vi "Test.vi"() -> ()   [LabVIEW 2017]
uses:
  libonnx_wrapper/libonnx_wrapper.lvlib
  postprocess_YOLOv8/postprocess_YOLOv8.lvlib
  libonnx_wrapper/TypeDef/IO.ctl
  libonnx_wrapper/TypeDef/Introspection.ctl
panel:
  out "Circles":cluster{"x":sgl, "y":sgl, "r":sgl}[](array[cluster])
  out "count":i32
  out "2D Picture":picture
  in  "BMP file path":path=path "/home/ivan/LabVIEWData/ONNX/LabVIEW_ONNX_YOLOv8/image_for_test/2005mmd_b2_1r_2005mmd_b2_var33.bmp"
  out "Metadata":string[][](table)
  out "Introspection Output":T1
  out "Introspection Input":T1
  in  "ONNX model path":path=path "/home/ivan/LabVIEWData/ONNX/LabVIEW_ONNX_YOLOv8/data/coins_detection.onnx"
  out "error out":errorcluster
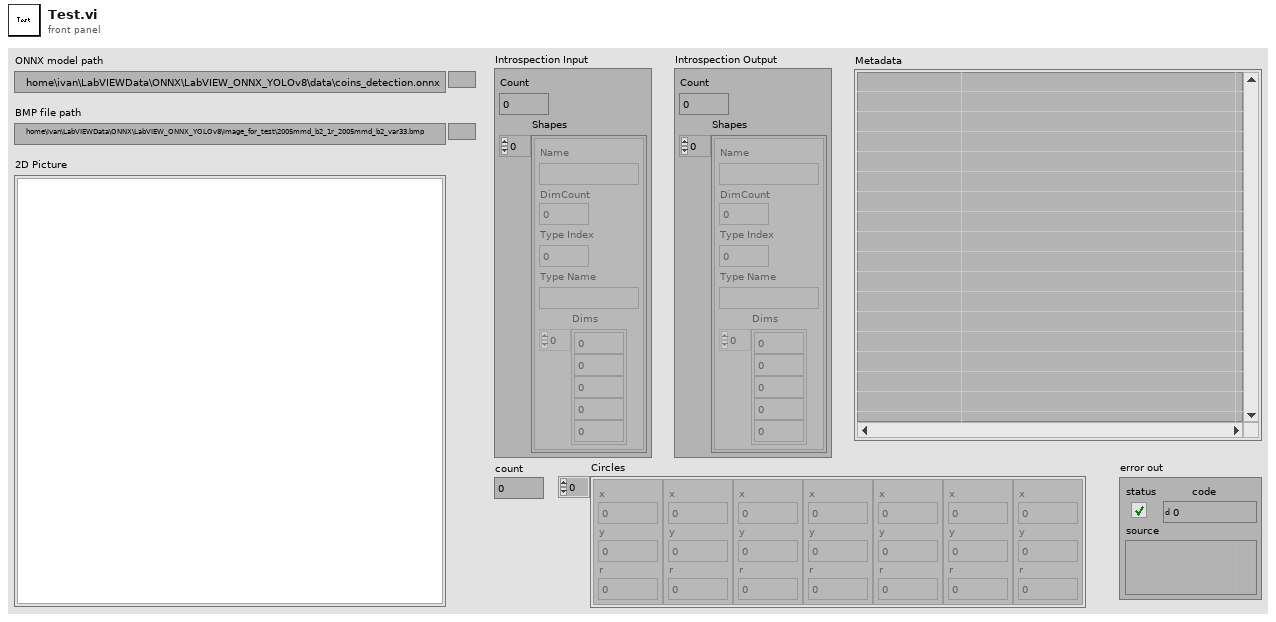
[diagram p1: front panel]
types:
  T1 = typedef "libonnx_wrapper.lvlib/Introspection.ctl" = cluster{"Count":i32, "Shapes":T2[]}
  T2 = typedef "libonnx_wrapper.lvlib/IO.ctl" = cluster{"Name":string, "DimCount":i32, "Type Index":i32, "Type Name":string, "Dims":i64[]}
  T3 = typedef "imagedata.ctl" = cluster{"image type":i32, "image depth":i32, "image":u8[], "mask":u8[], "colors":u32[], "Rectangle":cluster{"left":i16, "top":i16, "right":i16, "bottom":i16}}
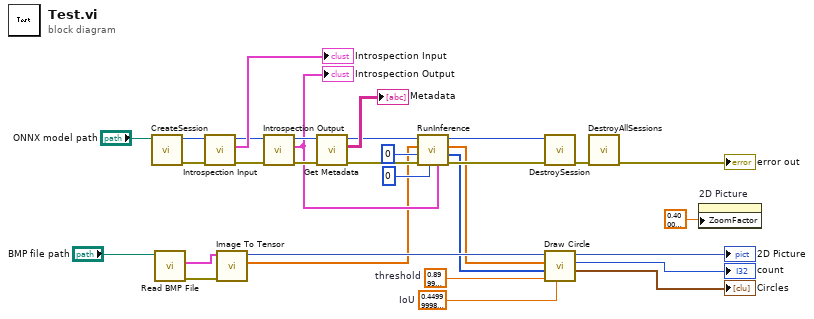
[diagram p0: block diagram]
diagram:
  w3 = sgl 0.45  # IoU
  w4 = sgl 0.9  # threshold
  n1 = call "CreateSession.vi"("ONNX model path"="ONNX model path") -> ("error out"=w14:errorcluster, "session id out"=w15:i32)  [unwired: 9 in]
  n2 = call <vilib>:"Read BMP File.vi"("path to BMP file"="BMP file path") -> ("error out"=w16:errorcluster, "image data"=w17:T3)  [unwired: 8 in, 1 out]
  n3 = call "Introspection Input.vi"("error in (no error)"=w14, "session id in"=w15) -> ("error out"=w27:errorcluster, "Introspection Input"=→"Introspection Input":T1, "session id out"=w28:i32)  [unwired: 7 in]
  n4 = call "Image To Tensor.vi"("error in (no error)"=w16, "image data"=w17) -> ("Data"=w7:sgl[], "image"=w11:picture)  [unwired: 7 in, 1 out]
  n5 = call "Introspection Output.vi"("error in (no error)"=w27, "session id in"=w28) -> ("error out"=w24:errorcluster, "Introspection Output"=w9:T1, "session id out"=w25:i32)  [unwired: 7 in]
  "Introspection Output" <- w9
  n6 = call "Get Metadata.vi"("error in (no error)"=w24, "session id in"=w25) -> ("error out"=w21:errorcluster, "Metadata"=→"Metadata":string[][], "session id out"=w22:i32)  [unwired: 7 in]
  n7 = call "RunInference.vi"("Introspection Output"=w9, "outputIndex"=0, "error in (no error)"=w21, "inputIndex"=0, "inputBuffer"=w7, "session id in"=w22) -> ("error out"=w13:errorcluster, "Dims"=w6:i64[], "outputBuffer"=w5:sgl[], "session id out"=w12:i32)  [unwired: 1 in, 1 out]
  n8 = call "DestroySession.vi"("error in (no error)"=w13, "session id in"=w12) -> ("error out"=w30:errorcluster)  [unwired: 8 in, 1 out]
  n9 = call "Draw Circle.vi"("IoU"=w3, "threshold"=w4, "dim"=w6, "data"=w5, "image in"=w11) -> ("Circles"=→"Circles":cluster{"x":sgl, "y":sgl, "r":sgl}[], "count"=→"count":i32, "image out"=→"2D Picture":picture)  [unwired: 4 in]
  n10 = call "DestroyAllSessions.vi"("error in (no error)"=w30) -> ("error out"=→"error out":errorcluster)  [unwired: 10 in]
  n11 = property on="2D Picture" class="Pict"("ZoomFactor"=sgl 0.4 ("Zoom Factor")) -> ()  [unwired: 2 in, 2 out]
